vi "multidimensional_ramp.vi"(3 "params":T1(array[cluster])) -> (0 "steps":i32, 1 "multidimensional ramp":dbl[][](array[numeric]))   [LabVIEW 2018]
doc: "MeasGUI - Measurement Graphics User Interface\nCopyright (c) 2018 Frans Korhonen\n\nMeasGUI was originally developed at Institute for Atmospheric \nand Earth System Research / Physics, Faculty of Science, \nUniversity of Helsinki, Finland\n\nAssistance, experience and feedback from following persons have been \ncritical in development of MeasGUI: Michel Attoui, Juha Kangasluoma, \nLauri Ahonen, Ella Häkkinen, Markku Kulmala and Tuukka Petäjä.\n\nThis file is part of MeasGUI.\n\nThis Source Code Form is subject to the terms of the Mozilla Public\nLicense, v. 2.0. If a copy of the MPL was not distributed with this\nfile, You can obtain one at http://mozilla.org/MPL/2.0/."
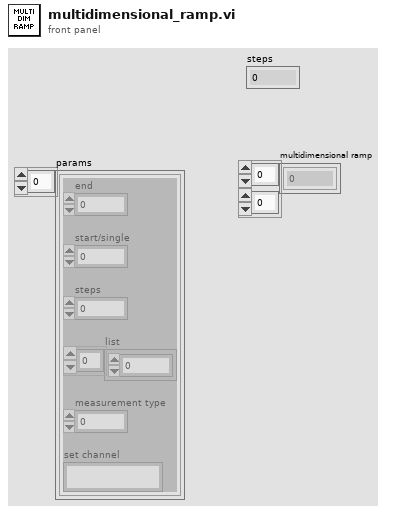
[diagram p1: front panel]
types:
  T1 = cluster{"end":dbl, "start/single":dbl, "steps":i32, "list":dbl[], "measurement type":u16, "set channel":string}[]
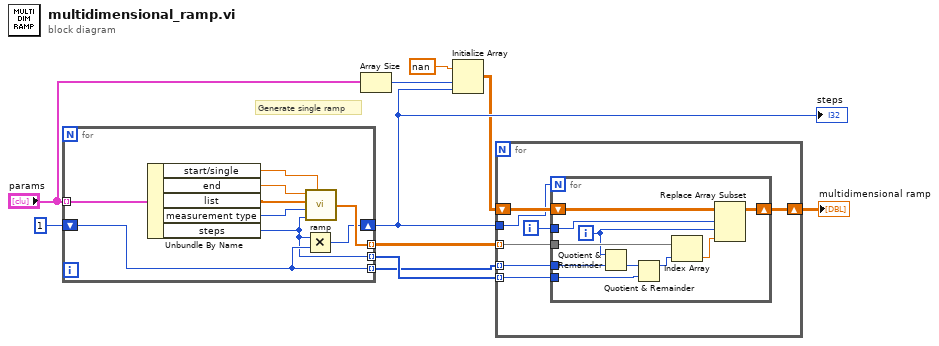
[diagram p0: block diagram]
diagram:
  # "Generate single ramp"
  n1 = for {
    tunnel: [w15] -> w4 mode=indexing
    shift-right: [w14] -> w8
    shift-left: 1 ("steps") -> [w12]
    tunnel: "params" -> [w13] mode=indexing
    tunnel: [w12] -> w5 mode=indexing
    tunnel: [w11] -> w10 mode=indexing
    n2 = Unbundle By Name(w13) -> ("start/single"=w19:dbl, "end"=w18:dbl, "list"=w17:dbl[], "measurement type"=w16:u16, "steps"=w11:i32)
    n3 = Multiply(x=w11, y=w12) -> (x*y=w14:i32)
    n4 = call "ramp.vi"("start /single"=w19, "Number of points"=w11, "Scan type"=w16, "chosen voltages"=w17, "end"=w18) -> ("values"=w15:dbl[])  [unwired: 1 out]
  }
  "steps" <- w8
  n5 = Array Size(array="params") -> (size(s)=w1:i32)
  n6 = Initialize Array(nan, w1, w8) -> (w7:dbl[][])
  n7 = for {
    tunnel: w4 -> [w26] mode=indexing
    shift-right: [w24] -> w9
    shift-left: w7 -> [w25]
    tunnel: w8 -> [w23]
    tunnel: w5 -> [w22] mode=indexing
    tunnel: w10 -> [w20] mode=indexing
    i -> [w21]
    n8 = for {
      N: w23 -> [_]
      tunnel: w26 -> [w35]
      tunnel: w21 -> [w29]
      shift-right: [w32] -> w24
      shift-left: w25 -> [w31]
      tunnel: w22 -> [w30]
      tunnel: w20 -> [w27]
      i -> [w28]
      n9 = Quotient & Remainder(x=w28, y=w30) -> (floor(x/y)=w36:i32)  [unwired: 1 out]
      n10 = Quotient & Remainder(x=w36, y=w27) -> (x-y*floor(x/y)=w34:i32)  [unwired: 1 out]
      n11 = Index Array(array=w35, index=w34) -> (element=w33:dbl)
      n12 = Replace Array Subset(array=w31, new element=w33, index (row)=w29, index (col)=w28) -> (w32:dbl[][])
    }
  }
  "multidimensional ramp" <- w9
